vi "Get Wire Terminals.vi"(8 "error in (no error)":errorcluster, 11 "Wire Refnum in":refnum<vi>) -> (0 "error out":errorcluster, 1 "Sink Terminals":refnum<vi>[](array[refnum]), 2 "Source Terminal":refnum<vi>, 3 "Wire Refnum out":refnum<vi>)   [LabVIEW 2018, in "Scripting.lvlib"]
uses:
  Scripting.lvlib
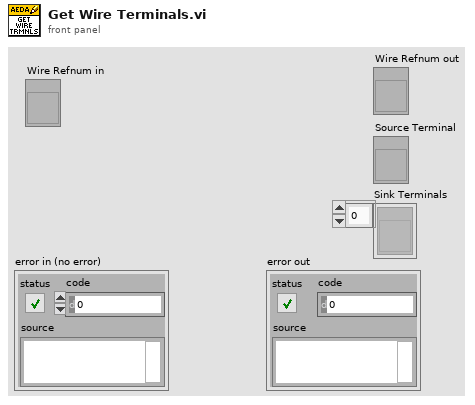
[diagram p1: front panel]
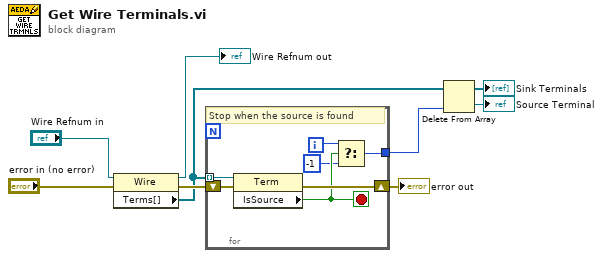
[diagram p0: block diagram]
diagram:
  n1 = property class="Wire"(reference="Wire Refnum in", error in="error in (no error)") -> (reference out=→"Wire Refnum out":refnum<vi>, error out=w7:errorcluster, "Terms[]"=w5:refnum<vi>[])
  n2 = for {
    tunnel: w5 -> [w15] mode=indexing
    shift-right: [w14] -> w4
    shift-left: w7 -> [w16]
    tunnel: [w10] -> w6
    i -> [w12]
    stop <- w13 stop-if-true
    # "Stop when the source is found"
    n3 = property class="Term"(reference=w15, error in=w16) -> (error out=w14:errorcluster, "IsSource"=w13:bool)  [unwired: 1 out]
    n4 = Select(t=w12, s=w13, f=-1) -> (s? t:f=w10:i32)
  }
  "error out" <- w4
  n5 = Delete From Array(array=w5, index=w6) -> (deleted portion=→"Source Terminal":refnum<vi>, array with subset deleted=→"Sink Terminals":refnum<vi>[])  [unwired: 1 in]
